vi "StartSequenceAcquisition.vi"(8 "error in (no error)":errorcluster, 10 "DataExchange":T1, 11 "Microscope in":refnum<class "Microscope.lvclass">) -> (0 "error out":errorcluster, 3 "Microscope out":refnum<class "Microscope.lvclass">)   [LabVIEW 2020, in "Microscope.lvlib" / "Microscope.lvclass"]
uses:
  Microscope.lvclass
  Component/Device/Device/DataExchange.ctl
  Hardware Layer/Real Hardware/Camera_Prime95B/Camera_Prime95B/Controls/Camera Status.ctl
  Hardware Layer/Real Hardware/Camera_Prime95B/Camera_Prime95B/Controls/AcquisitionParams.ctl
  Microscope.lvclass/Microscope.ctl
  Component/Device/Device Messages/StartSequenceAcquisition Msg/StartSequenceAcquisition Msg.lvclass/StartSequenceAcquisition Msg.ctl
  <vilib>/ActorFramework/Message Enqueuer/Message Enqueuer.lvclass/Message Enqueuer.ctl
  Logic Layer/DataLogger/DataLogger Messages/StartLogging Msg/StartLogging Msg.lvclass/StartLogging Msg.ctl
  <vilib>/ActorFramework/Message Enqueuer/Enqueue.vi
  Component/Device/Device Messages/StartSequenceAcquisition Msg/StartSequenceAcquisition Msg.lvclass
  C:/Program Files/National Instruments/LabVIEW 2020/vi.lib/ActorFramework/Message/Message.lvclass
  Logic Layer/DataLogger/DataLogger Messages/StartLogging Msg/StartLogging Msg.lvclass
  <vilib>/ActorFramework/Message Priority Queue/Priority Enqueue.vi
  Component/Device/Device/Device.lvclass
  Hardware Layer/Real Hardware/Camera_Prime95B/Camera_Prime95B/Camera_Prime95B.lvclass
  Interface/DataListener/DataListener.lvclass
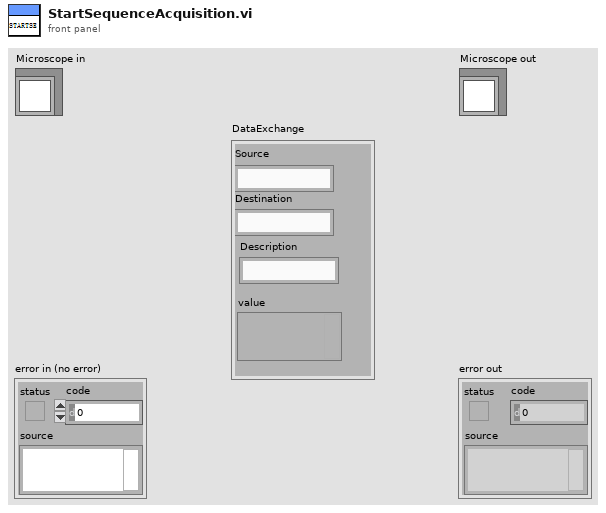
[diagram p1: front panel]
types:
  T1 = typedef "DataListener.lvclass/DataExchange.ctl" = cluster{"Source":string, "Destination":string, "Description":string, "value":variant}
  T2 = typedef "Camera_Prime95B.lvlib/Camera_Prime95B.lvclass/Camera Status.ctl" = i32
  T3 = typedef "Camera_Prime95B.lvlib/Camera_Prime95B.lvclass/AcquisitionParams.ctl" = cluster{"Acq Mode":T2, "Save Path":path, "Stream Save Path":path, "SingleStack?":bool, "StreamToDisk?":bool, "Alert when finish?":bool}
  T4 = map{string, refnum<class "Message Enqueuer.lvclass">}
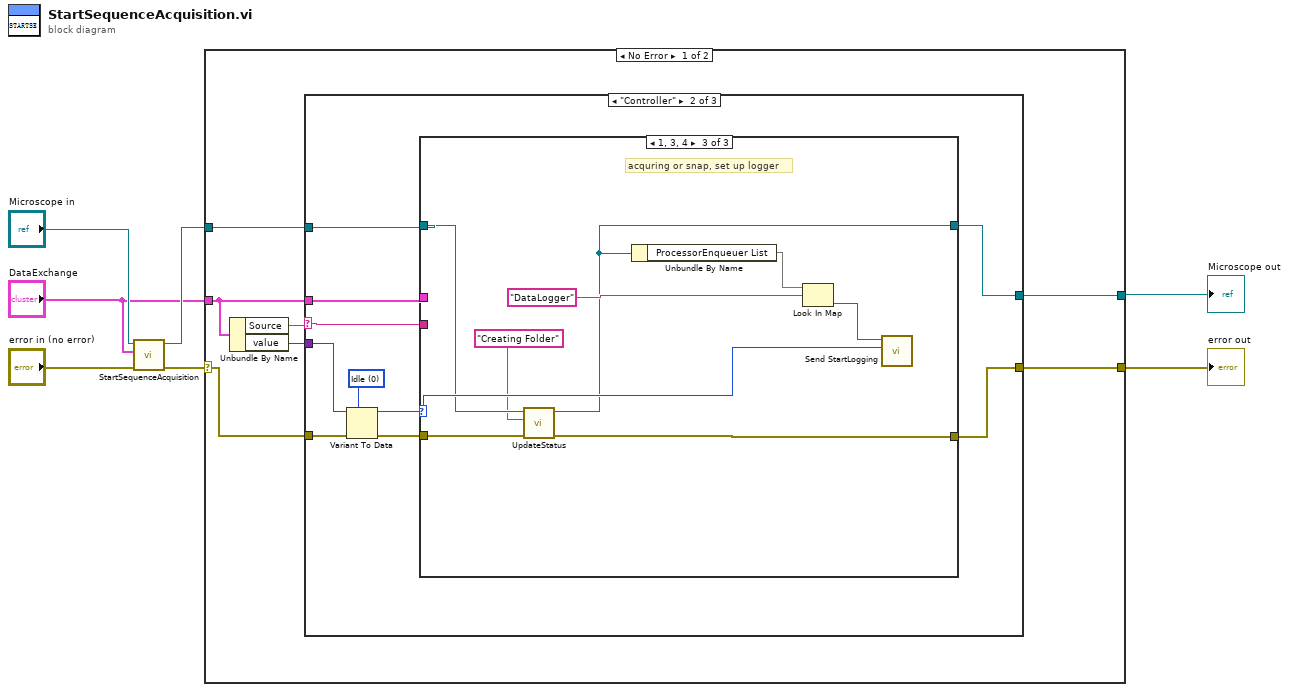
[diagram p0: block diagram]
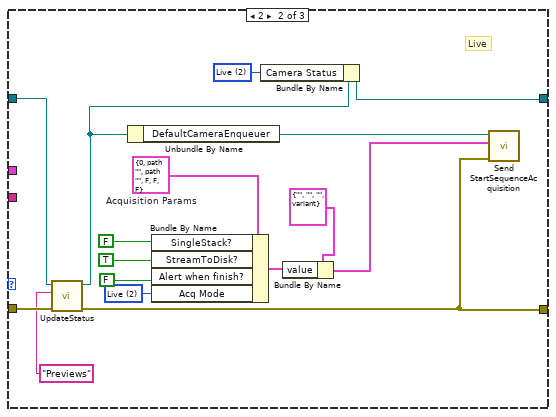
[diagram p4: hidden frame]
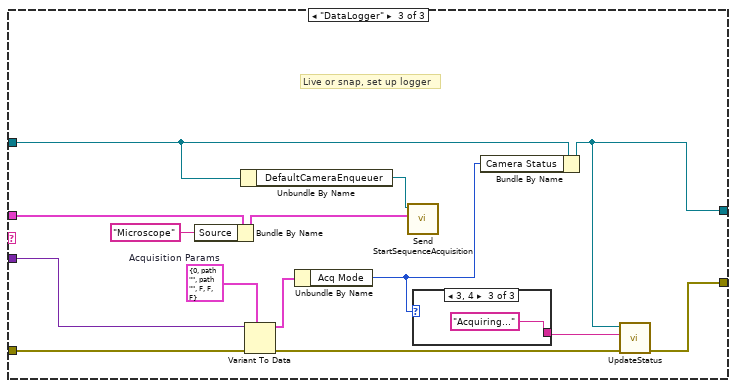
[diagram p5: hidden frame]
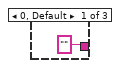
[diagram p6: hidden frame]
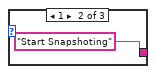
[diagram p7: hidden frame]
diagram:
  n1 = call-parent "StartSequenceAcquisition.vi"("error in (no error)"="error in (no error)", "DataExchange"="DataExchange", "Device in"="Microscope in") -> ("error out"=w5:errorcluster, "Device out"=w3:refnum<class "Microscope.lvclass">)  [unwired: 7 in]
  n2 = case shown="No Error" w5 {
    selector: w5 -> [w14 w71]
    tunnel: [w10 w71] -> w4
    tunnel: [w11 w72] -> w2
    tunnel: w3 -> [w12 w72]
    tunnel: "DataExchange" -> [w9 _]
    frame No Error {
      n3 = Unbundle By Name(w9) -> ("Source"=w8:string, "value"=w13:variant)
      n4 = case shown="\"Controller\"" w8 {
        selector: w8 -> [_ w17 _]
        tunnel: w14 -> [w15 w26 w67]
        tunnel: w13 -> [_ w24 w58]
        tunnel: w12 -> [w16 w21 w61]
        tunnel: [w16 w20 w55] -> w11
        tunnel: [w15 w19 w62] -> w10
        tunnel: w9 -> [_ w18 w66]
        frame Default {
        }
        frame "Controller" {
          w23 = T2 0 items=["Idle", "Snap", "Live", "Capturing", ""] ("Mode")
          n5 = Variant To Data(error in=w26, type=w23, Variant=w24) -> (data=w22:T2, error out=w25:errorcluster)
          n6 = case shown="1, 3, 4" w22 {
            selector: w22 -> [_ _ w50]
            tunnel: w25 -> [w28 w43 w49]
            tunnel: [w28 w34 w48] -> w19
            tunnel: w21 -> [w27 w33 w47]
            tunnel: [w27 w30 w46] -> w20
            tunnel: w18 -> [_ _ _]
            tunnel: w17 -> [_ _ _]
            frame 0, Default {
            }
            frame 2 {
              w29 = T2 2 items=["Idle", "Snap", "Live", "Capturing", ""] ("Camera Status")
              w35 = T2 2 items=["Idle", "Snap", "Live", "Capturing", ""] ("Acq Mode")
              w42 = T3 {"Acq Mode"=0, "Save Path"=path "", "Stream Save Path"=path "", "SingleStack?"=FALSE, "StreamToDisk?"=FALSE, "Alert when finish?"=FALSE}  # Acquisition Params
              # "Live"
              n7 = call-dynamic "UpdateStatus.vi"("error in (no error)"=w43, "Description"="Previews", "Microscope in"=w33) -> ("error out"=w34:errorcluster, "Microscope out"=w32:refnum<class "Microscope.lvclass">)  [unwired: 7 in]
              n8 = Unbundle By Name(w32) -> ("DefaultCameraEnqueuer"=w44:refnum<class "Message Enqueuer.lvclass">)
              n9 = Bundle By Name(cluster=w42, "SingleStack?"=FALSE, "StreamToDisk?"=TRUE, "Alert when finish?"=FALSE, "Acq Mode"=w35) -> (w41:T3)
              n10 = Bundle By Name(cluster=w32, "Camera Status"=w29) -> (w30:refnum<class "Microscope.lvclass">)
              n11 = Bundle By Name(cluster=T1 {"Source"="", "Destination"="", "Description"="", "value"=variant} ("input cluster"), "value"=w41) -> (w36:T1)
              n12 = call "Send StartSequenceAcquisition.vi"("error in (no error)"=w34, "DataExchange"=w36, "Message Enqueuer"=w44) -> ()  [unwired: 7 in, 2 out]
            }
            frame 1, 3, 4 {
              # "acquring or snap, set up logger"
              n13 = call-dynamic "UpdateStatus.vi"("error in (no error)"=w49, "Description"="Creating Folder", "Microscope in"=w47) -> ("error out"=w48:errorcluster, "Microscope out"=w46:refnum<class "Microscope.lvclass">)  [unwired: 7 in]
              n14 = Unbundle By Name(w46) -> ("ProcessorEnqueuer List"=w53:T4)
              n15 = Look In Map(map=w53, key="DataLogger") -> (value=w51:refnum<class "Message Enqueuer.lvclass">)  [unwired: 1 in, 1 out]
              n16 = call "Send StartLogging.vi"("Mode"=w50, "Message Enqueuer"=w51) -> ()  [unwired: 8 in, 2 out]
            }
          }
        }
        frame "DataLogger" {
          w57 = T3 {"Acq Mode"=0, "Save Path"=path "", "Stream Save Path"=path "", "SingleStack?"=FALSE, "StreamToDisk?"=FALSE, "Alert when finish?"=FALSE}  # Acquisition Params
          # "Live or snap, set up logger"
          n17 = Bundle By Name(cluster=w66, "Source"="Microscope") -> (w64:T1)
          n18 = Unbundle By Name(w61) -> ("DefaultCameraEnqueuer"=w65:refnum<class "Message Enqueuer.lvclass">)
          n19 = Variant To Data(error in=w67, type=w57, Variant=w58) -> (data=w56:T3, error out=w59:errorcluster)
          n20 = Unbundle By Name(w56) -> ("Acq Mode"=w54:T2)
          n21 = call "Send StartSequenceAcquisition.vi"("DataExchange"=w64, "Message Enqueuer"=w65) -> ()  [unwired: 8 in, 2 out]
          n22 = case shown="3, 4" w54 {
            tunnel: ["" ("Description") "Start Snapshoting" ("Description") "Acquiring..." ("Description")] -> w60
            frame 0, Default {
            }
            frame 1 {
            }
            frame 3, 4 {
            }
          }
          n23 = Bundle By Name(cluster=w61, "Camera Status"=w54) -> (w55:refnum<class "Microscope.lvclass">)
          n24 = call-dynamic "UpdateStatus.vi"("error in (no error)"=w59, "Description"=w60, "Microscope in"=w55) -> ("error out"=w62:errorcluster)  [unwired: 7 in, 1 out]
        }
      }
    }
    frame Error {
    }
  }
  "error out" <- w4
  "Microscope out" <- w2
